vi "solve NNLS LV.vi"(4 "data Matrix Szie":T1, 5 "D":dbl[](array[numeric]), 6 "fIRF":dbl[](array[numeric]), 7 "vv":dbl[](array[numeric]), 8 "error in (no error)":errorcluster, 9 "RHS_multiplier_array":dbl[](array[numeric]), 10 "LHS_multiplier_array":dbl[](array[numeric]), 11 "LCs":dbl[](array[numeric])) -> (0 "error out":errorcluster, 1 "LC_rows out":u64, 2 "LC_cols out":u64, 3 "LCs out":dbl[](array[numeric]))   [LabVIEW 2024, in "LaguerreDeconLib.lvlib"]
doc: "extern \"C\" DECONLIBRARY_API void solveNNLS_LV(double* LHS_multiplier_array, unsigned long long LHSrows, unsigned long long LHScols,\n double* fIRF, unsigned long long length,\n double* RHS_multiplier_array, unsigned long long RHSrows, unsigned long long RHScols,\n double* vv, unsigned long long vvRows, unsigned long long vvCols,\n double* D, unsigned long long DRows, unsigned long long DCols,\n double* LCs, unsigned long long* LC_rows, unsigned long long* LC_cols);"
uses:
  LaguerreDeconLib.lvlib
  LaguerreDeconDLL.dll
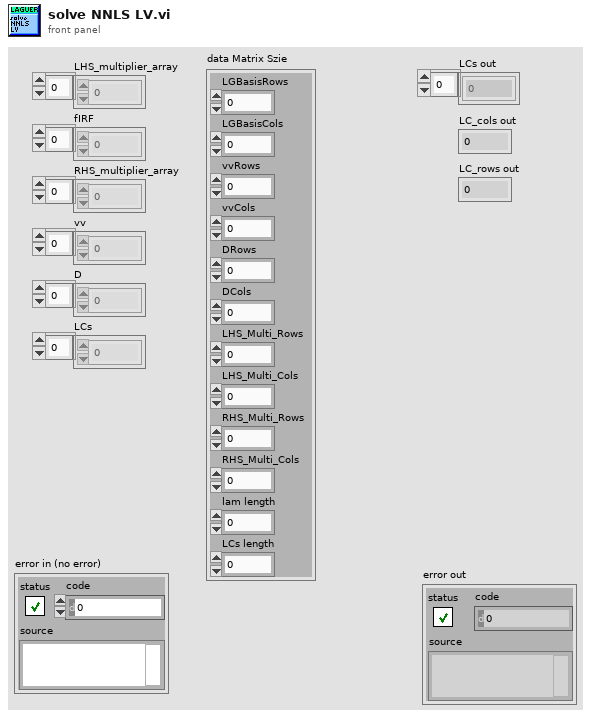
[diagram p1: front panel]
types:
  T1 = cluster{"LGBasisRows":u64, "LGBasisCols":u64, "vvRows":u64, "vvCols":u64, "DRows":u64, "DCols":u64, "LHS_Multi_Rows":u64, "LHS_Multi_Cols":u64, "RHS_Multi_Rows":u64, "RHS_Multi_Cols":u64, "lam length":u64, "LCs length":u64}
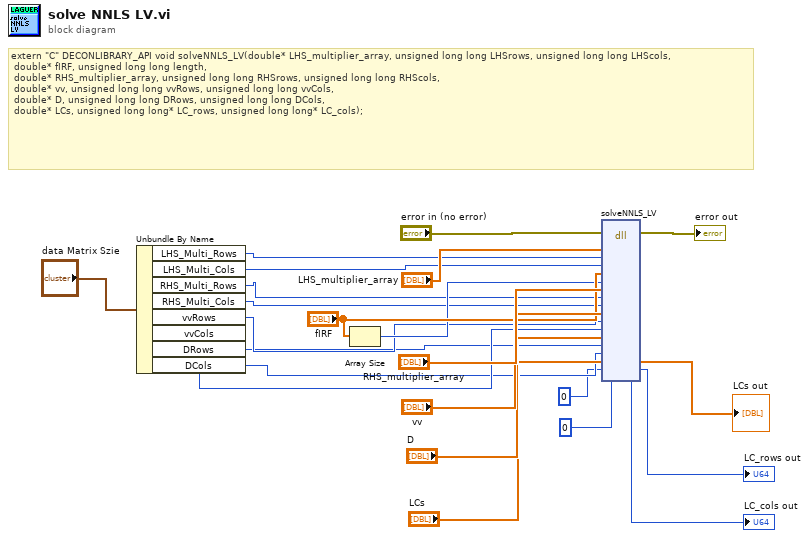
[diagram p0: block diagram]
diagram:
  # "extern \"C\" DECONLIBRARY_API void solveNNLS_LV(double* LHS_multiplier_array, unsigned long long LHSrows, unsigned long long LHScols,\n\tdouble* fIRF, unsigned long long length,\n\tdouble* RHS_multiplier_array, unsigned long long RHSrows, unsigned long long RHScols,\n\tdouble* vv, unsigned long long vvRows, unsigned long long vvCols,\n\tdouble* D, unsigned long long DRows, unsigned long long DCols,\n\tdouble* LCs, unsigned long long* LC_rows, unsigned long long* LC_cols);"
  n1 = Unbundle By Name("data Matrix Szie") -> ("LHS_Multi_Rows"=w14:u64, "LHS_Multi_Cols"=w13:u64, "RHS_Multi_Rows"=w10:u64, "RHS_Multi_Cols"=w9:u64, "vvRows"=w8:u64, "vvCols"=w7:u64, "DRows"=w6:u64, "DCols"=w5:u64)
  n2 = Array Size(array="fIRF") -> (size(s)=w11:i32)
  n3 = dll-call lib="C:/Users/MarcuLab/Desktop/V6 APD LV/V6 APD LV/LaguerreDeconLib/LaguerreDeconDLL.dll" fn="solveNNLS_LV"(error in="error in (no error)", "LHS_multiplier_array"="LHS_multiplier_array", "LHSrows"=w14, "LHScols"=w13, "fIRF"="fIRF", "length"=w11, "RHS_multiplier_array"="RHS_multiplier_array", "RHSrows"=w10, "RHScols"=w9, "vv"="vv", "vvRows"=w8, "vvCols"=w7, "D"="D", "DRows"=w6, "DCols"=w5, "LCs"="LCs", "LC_rows"=u64 0, "LC_cols"=u64 0) -> (error out=→"error out":errorcluster, "LCs"=→"LCs out":dbl[], "LC_rows"=→"LC_rows out":u64, "LC_cols"=→"LC_cols out":u64)  [unwired: 17 in, 1 out]
